vi "Update Alias name.vi"(8 "error in (no error)":errorcluster, 9 "New Alias name":string, 10 "Alias":string, 11 "Aliases Ref in":T1 format="%.0x") -> (0 "error out":errorcluster, 3 "Aliases Ref out":T1 format="%.0x")   [LabVIEW 2017, in "SLSC Switch Scripting.lvlib"]
uses:
  SLSC Switch Scripting.lvlib
  <vilib>/NI Veristand/Custom Device API/Custom Device Item Ref.ctl
  <vilib>/NI Veristand/Custom Device API/Set Item Property (String).vi
  <vilib>/NI VeriStand/Custom Device API/Custom Device API.lvlib
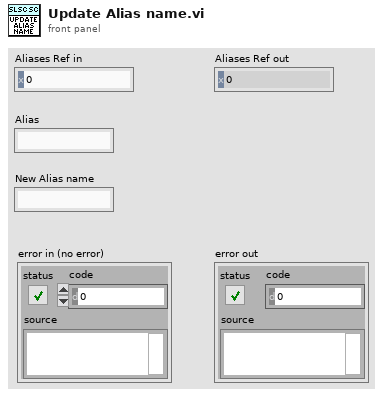
[diagram p1: front panel]
types:
  T1 = typedef "Custom Device API.lvlib/Custom Device Item Ref.ctl" = u64
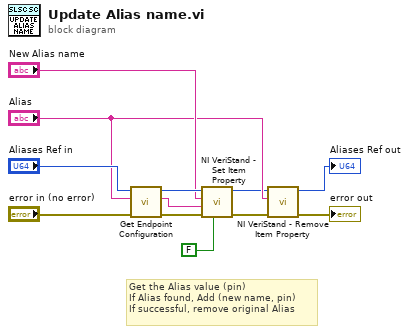
[diagram p0: block diagram]
diagram:
  # "Get the Alias value (pin)\nIf Alias found, Add (new name, pin)\nIf successful, remove original Alias"
  n1 = call "Get Endpoint Configuration.vi"("error in (no error)"="error in (no error)", "Alias"="Alias", "Aliases Ref in"="Aliases Ref in") -> ("error out"=w7:errorcluster, "Pin"=w8:string, "Aliases Ref out"=w10:T1)  [unwired: 5 in, 1 out]
  n2 = call-poly <vilib>:"NI VeriStand - Set Item Property.vi"("Binary String (T)"=FALSE, "error in (no error)"=w7, "Value"=w8, "Property Name"="New Alias name", "Item Ref in"=w10) -> ("error out"=w2:errorcluster, "Item Ref out"=w1:T1)  [unwired: 4 in, 1 out]
  n3 = call <vilib>:"NI VeriStand - Remove Item Property.vi"("error in (no error)"=w2, "Property Name"="Alias", "Item Ref in"=w1) -> ("error out"=→"error out":errorcluster, "Item Ref out"=→"Aliases Ref out":T1)  [unwired: 6 in, 1 out]
